vi "Write Size.vi"(5 "Size":T1, 9 "Path in":refnum<class "Path.lvclass">) -> (3 "Path out":refnum<class "Path.lvclass">)   [LabVIEW 2014, in "Path.lvclass"]
uses:
  Path.lvclass
  <vilib>/Utility/miscctls.llb/LVBoundsTypeDef.ctl
  Path.lvclass/Path.ctl
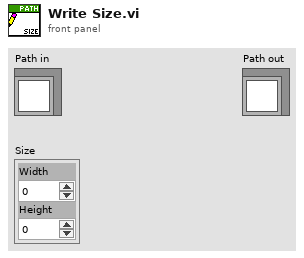
[diagram p1: front panel]
types:
  T1 = typedef "LVBoundsTypeDef.ctl" = cluster{"Width":u32, "Height":u32}
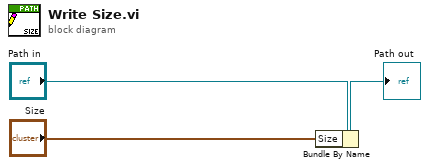
[diagram p0: block diagram]
diagram:
  n1 = Bundle By Name(cluster="Path in", "Size"="Size") -> (→"Path out":refnum<class "Path.lvclass">)
